vi "Flatten to MessageString.vi"(8 "error in (no error)":errorcluster, 10 "Message Priority":T1=enum."Normal", 11 "Actor Framework:Message":refnum<class "Message.lvclass">) -> (0 "error out":errorcluster, 3 "Msg String":T2={"Flatten Msg"="", "Message Priority"=enum."Normal"})   [LabVIEW 2014, in "Network Stream.lvlib" / "Network Stream.lvclass"]
uses:
  Network Stream.lvclass
  MessageString.ctl
  <vilib>/ActorFramework/Message Enqueuer/Message Priority.ctl
  <vilib>/ActorFramework/Message/Message.lvclass
  <vilib>/ActorFramework/Message Enqueuer/Message Enqueuer.lvclass
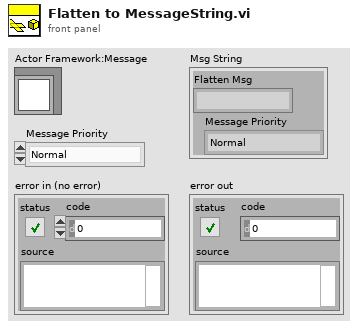
[diagram p1: front panel]
types:
  T1 = typedef "Actor Framework.lvlib/Message Enqueuer.lvclass/Message Priority.ctl" = enum16{"Low", "Normal", "High"}
  T2 = typedef "Network Stream.lvlib/Network Stream.lvclass/MessageString.ctl" = cluster{"Flatten Msg":string, "Message Priority":T1}
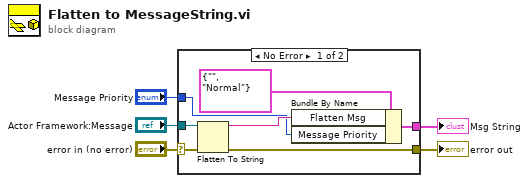
[diagram p0: block diagram]
diagram:
  n1 = case shown="No Error" "error in (no error)" {
    selector: "error in (no error)" -> [w6 w13]
    tunnel: [w11 _] -> w5
    tunnel: "Actor Framework:Message" -> [w9 _]
    tunnel: [w8 w13] -> w3
    tunnel: "Message Priority" -> [w7 _]
    frame No Error {
      n2 = Flatten To String(anything=w9, error in (no error)=w6) -> (data string=w10:string, error out=w8:errorcluster)  [unwired: 2 in, 1 out]
      n3 = Bundle By Name(cluster=T2 {"Flatten Msg"="", "Message Priority"=enum."Normal"} ("Msg String"), "Flatten Msg"=w10, "Message Priority"=w7) -> (w11:T2)
    }
    frame Error {
    }
  }
  "Msg String" <- w5
  "error out" <- w3
